vi "UI Style.vi"() -> ()   [LabVIEW 2023, in "VIDoc Parsing.lvlib" / "Structure Reporter.lvlib"]
uses:
  Structure Reporter.lvlib
  <vilib>/platform/TimedLoop/XDataNode/XDataNode.xnode
  <vilib>/Platform/TimedLoop/XDataNode/nitl_modes.ctl
  <vilib>/Platform/TimedLoop/XDataNode/XDNodeRunTimeDep.lvlib
  <vilib>/Platform/TimedLoop/XDataNode/wakeup.ctl
  <vilib>/Platform/TimedLoop/XDataNode/timing_clust.ctl
panel:
  in  "stop":bool
  in  "OK Button":bool
  in  "Boolean":bool
  in  "Numeric":dbl
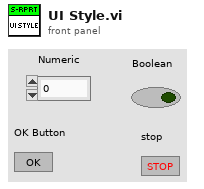
[diagram p1: front panel]
types:
  T1 = typedef "XDNodeRunTimeDep.lvlib/timing_clust.ctl" = cluster{"Expected End [f-1]":u64, "Actual End [f-1]":u64, "Finished Late? [f-1]":bool, "Expected End [i-1]":u64, "Actual End [i-1]":u64, "Finished Late? [i-1]":bool, "Expected Start [i]":u64, "Actual Start [i]":u64, "Expected Start [f]":u64, "Actual Start [f]":u64, "Source Name":string, "Structure Name":string, "Period":i64, "Deadline":i64, "Offset":i64, "Start":i64, "Priority":i32, "Timeout":i32, "Mode":T2, "Wakeup Reason":T3, "Error":errorcluster, "Source Type":string, "Secondary Source Type":string, "Global End Time":u64, "Global Start Time":u64, "Frame Duration":u64, "Iteration Duration":u64, "Assigned CPU":i32, "I/O Scan Engine Mode":u32}
  T2 = typedef "XDNodeRunTimeDep.lvlib/nitl_modes.ctl" = enum32{"No Change", "Process missed periods, maintain original phase", "Discard missed periods, maintain original phase", "Process missed periods, ignore original phase", "Discard missed periods, ignore original phase"}
  T3 = typedef "XDNodeRunTimeDep.lvlib/wakeup.ctl" = enum32{"Normal", "Aborted", "Asynchronous wakeup", "Timing source error", "Timed loop error", "Timeout"}
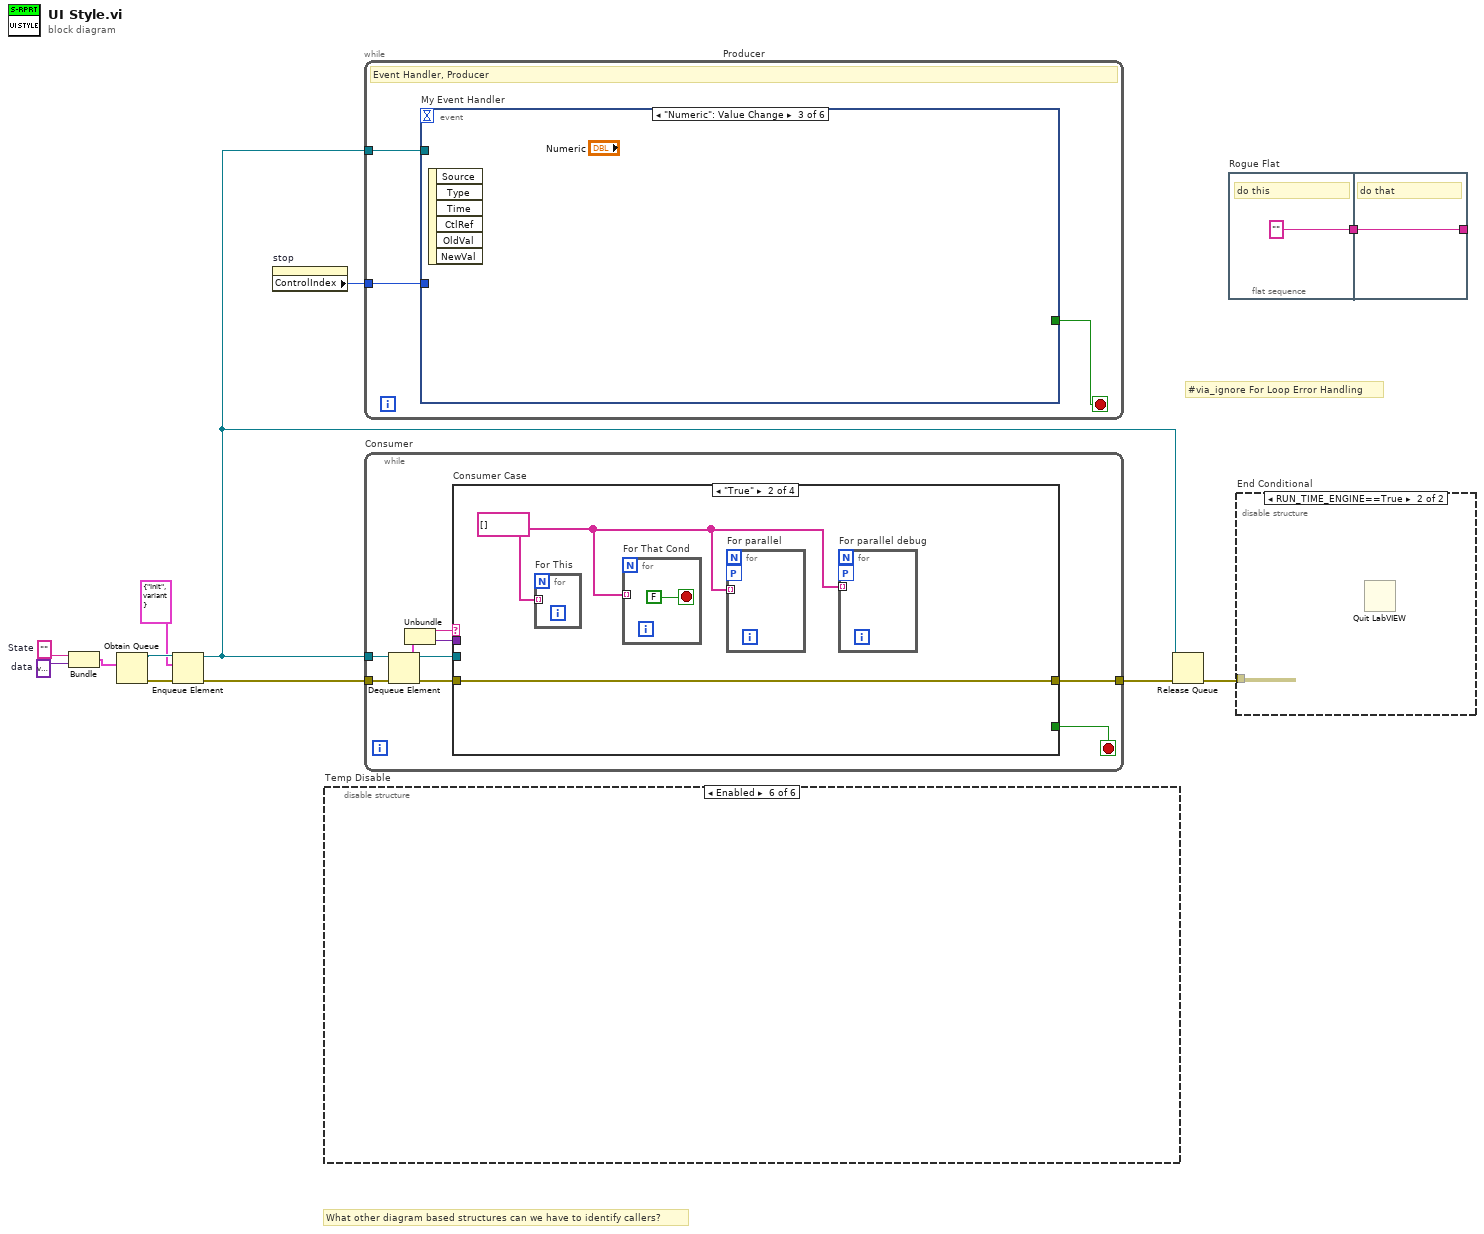
[diagram p0: block diagram]
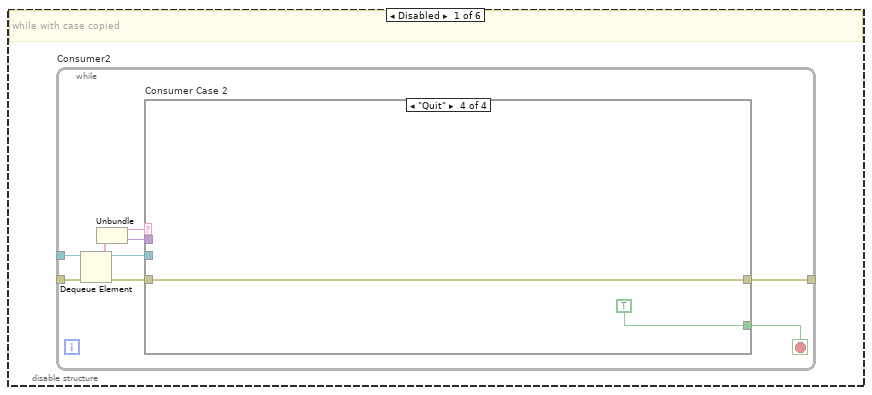
[diagram p3: hidden frame]
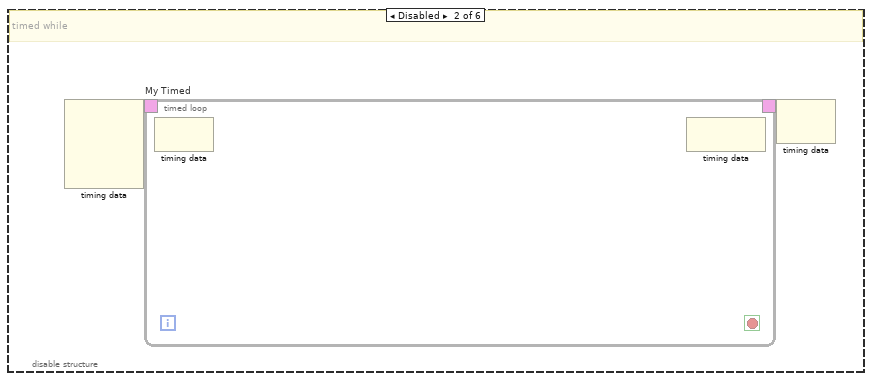
[diagram p7: hidden frame]
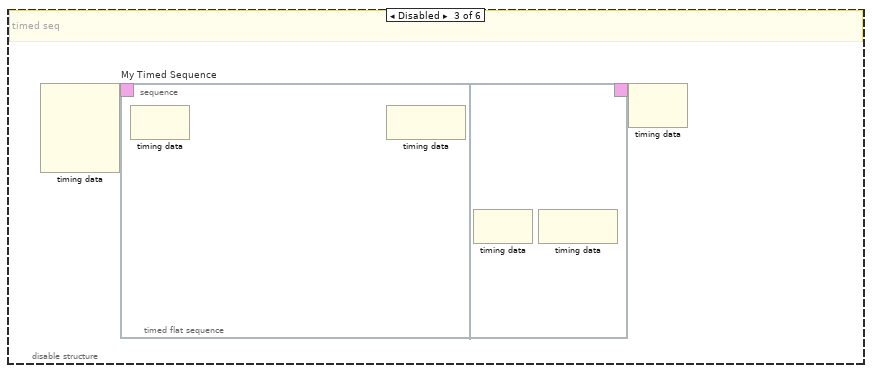
[diagram p8: hidden frame]
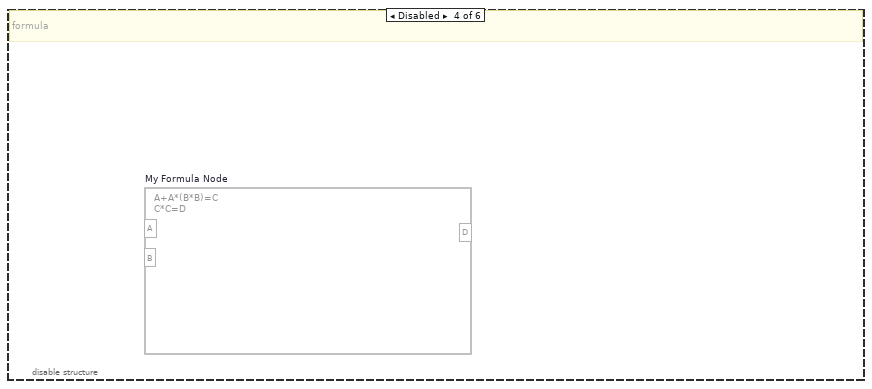
[diagram p9: hidden frame]
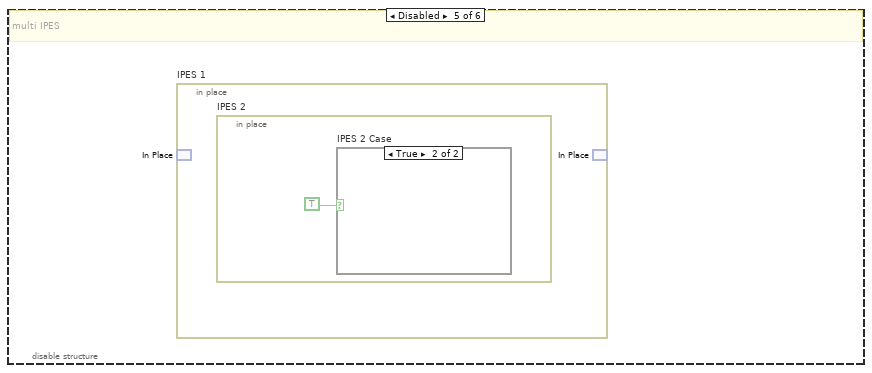
[diagram p10: hidden frame]
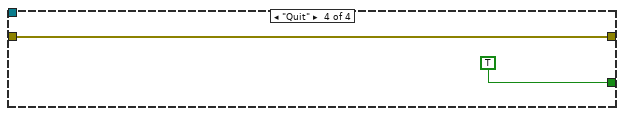
[diagram p14: hidden frame]
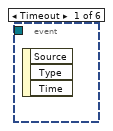
[diagram p15: hidden frame]
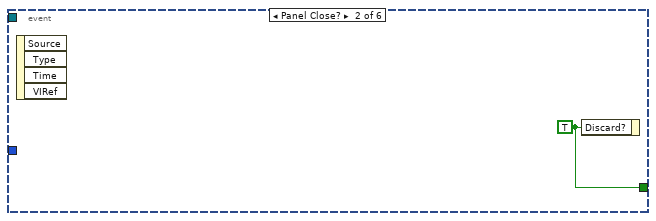
[diagram p16: hidden frame]
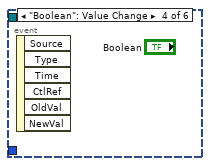
[diagram p17: hidden frame]
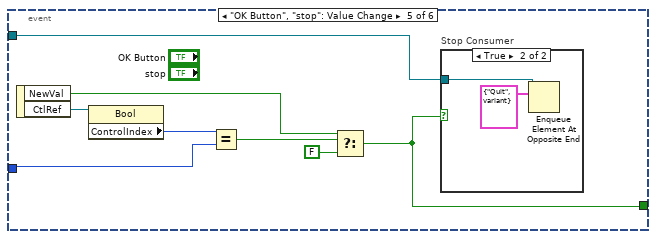
[diagram p18: hidden frame]
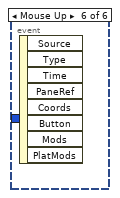
[diagram p20: hidden frame]
diagram:
  w11 = variant  # data
  w12 = ""  # State
  # "#via_ignore For Loop Error Handling"
  # "What other diagram based structures can we have to identify callers?"
  n1 = Bundle("State"=w12, "data"=w11) -> (w10:cluster{"State":string, "data":variant})  [unwired: 1 in]
  n2 = Obtain Queue(element data type=w10) -> (queue out=w9:refnum<queue>, error out=w7:errorcluster)  [unwired: 4 in, 1 out]
  n3 = Enqueue Element(queue=w9, element=cluster{"State":string, "data":variant} {"State"="Init", "data"=variant}, error in (no error)=w7) -> (queue out=w5:refnum<queue>, error out=w8:errorcluster)  [unwired: 1 in, 1 out]
  n4 = property on="stop" class="Bool"() -> ("ControlIndex"=w3:i32)  [unwired: 2 in, 2 out]
  n5 = disable-structure "Temp Disable" shown="Enabled" {
    frame Disabled {
      # "while with case copied"
      n6 = while "Consumer2" {
        tunnel: _ -> [w21]
        tunnel: _ -> [w15]
        tunnel: [w14] -> _
        stop <- w13 stop-if-true
        n7 = Dequeue Element(queue=w21, error in (no error)=w15) -> (queue out=w17:refnum<queue>, element=w20:cluster{"State":string, "data":variant}, error out=w16:errorcluster)  [unwired: 1 in, 1 out]
        n8 = Unbundle(w20) -> ("State"=w19:string, "data"=w18:variant)
        n9 = case "Consumer Case 2" shown="\"Quit\"" w19 {
          tunnel: w18 -> [_ _ _ _]
          tunnel: w17 -> [_ _ _ _]
          tunnel: w16 -> [w22 w23 w24 w29]
          tunnel: [w22 w23 w26 w29] -> w14
          tunnel: [_ _ _ TRUE] -> w13
          frame "False", Default {
          }
          frame "True" {
          }
          frame "Init" {
            n10 = flat-sequence "Init Flat 2" {
              tunnel: [w27] -> w25
              tunnel: w24 -> [w27]
              tunnel: [w28] -> w26
              tunnel: w25 -> [w28]
              frame #0 {
                # "do this"
              }
              frame #1 {
                # "do that"
              }
            }
          }
          frame "Quit" {
          }
        }
      }
    }
    frame Disabled {
      # "timed while"
      n11 = node-c288() -> (w32:T1)  [unwired: 4 in]
      n12 = timed-loop "My Timed" {
        timing: w32 -> [_]
        timing-out: [_] -> w31
        stop <- _ stop-if-true
        n13 = node-c288() -> ()  [unwired: 1 in, 1 out]
        n14 = node-c288() -> ()  [unwired: 1 in, 1 out]
      }
      n15 = node-c288(w31) -> ()  [unwired: 1 out]
    }
    frame Disabled {
      # "timed seq"
      n16 = node-c288() -> (w38:T1)  [unwired: 4 in]
      n17 = timed-sequence "My Timed Sequence" {
        timing: w38 -> [_]
        timing-out: [_] -> w37
        n18 = timed-flat-sequence {
          frame #0 {
            n19 = node-c288() -> ()  [unwired: 1 in, 1 out]
            n20 = node-c288() -> ()  [unwired: 1 in, 1 out]
          }
          frame #1 {
            n21 = node-c288() -> ()  [unwired: 1 in, 1 out]
            n22 = node-c288() -> ()  [unwired: 1 in, 1 out]
          }
        }
      }
      n23 = node-c288(w37) -> ()  [unwired: 1 out]
    }
    frame Disabled {
      # "formula"
      n24 = formula code="A+A*(B*B)=C\nC*C=D" "My Formula Node"() -> ()  [unwired: 2 in, 1 out]
    }
    frame Disabled {
      # "multi IPES"
      n25 = in-place "IPES 1" {
        n26 = in-place-match #1() -> ()  [unwired: 1 in, 1 out]
        n27 = in-place "IPES 2" {
          n28 = case "IPES 2 Case" shown="True" TRUE {
            frame False {
            }
            frame True {
            }
          }
        }
        n29 = in-place-match #1() -> ()  [unwired: 1 in, 1 out]
      }
    }
    frame Enabled {
    }
  }
  n30 = while "Producer" {
    tunnel: w5 -> [w47]
    tunnel: w3 -> [w46]
    stop <- w48 stop-if-true
    # "Event Handler, Producer"
    n31 = event "My Event Handler" shown="[2] \"Numeric\": Value Change" {
      selector: _ -> [_ _ _ _ _ _]
      dyn-events: _ -> [_ _ _ _ _ _]
      timeout: _ -> [_ _ _ _ _ _]
      tunnel: [_ w49 _ _ w51 _] -> w48
      tunnel: w47 -> [_ _ _ _ w50 _]
      tunnel: w46 -> [_ _ _ _ w55 _]
      event Timeout {
        n32 = event-data() -> ()  [unwired: 1 in, 3 out]
      }
      event Panel Close? {
        w49 = TRUE ("Discard?")
        n33 = event-data() -> ()  [unwired: 1 in, 4 out]
        n34 = event-data("Discard?"=w49) -> ()  [unwired: 1 in, 1 out]
      }
      event "Numeric": Value Change {
        n35 = event-data() -> ()  [unwired: 1 in, 6 out]
      }
      event "Boolean": Value Change {
        n36 = event-data() -> ()  [unwired: 1 in, 6 out]
      }
      event "OK Button", "stop": Value Change {
        n37 = event-data() -> ("NewVal"=w53:bool, "CtlRef"=w57:refnum<vi>)  [unwired: 1 in]
        n38 = property class="Bool"(reference=w57) -> ("ControlIndex"=w56:i32)  [unwired: 1 in, 2 out]
        n39 = Equal?(x=w56, y=w55) -> (x = y?=w54:bool)
        n40 = Select(t=w53, s=w54, f=FALSE) -> (s? t:f=w51:bool)
        n41 = case "Stop Consumer" shown="True" w51 {
          tunnel: w50 -> [_ w59]
          frame False {
          }
          frame True {
            n42 = Enqueue Element At Opposite End(queue=w59, element=cluster{"State":string, "data":variant} {"State"="Quit", "data"=variant}) -> ()  [unwired: 2 in, 3 out]
          }
        }
      }
      event Mouse Up {
        n43 = event-data() -> ()  [unwired: 1 in, 8 out]
      }
    }
  }
  n44 = while "Consumer" {
    tunnel: w5 -> [w68]
    tunnel: w8 -> [w62]
    tunnel: [w61] -> w6
    stop <- w60 stop-if-true
    n45 = Dequeue Element(queue=w68, error in (no error)=w62) -> (queue out=w64:refnum<queue>, element=w67:cluster{"State":string, "data":variant}, error out=w63:errorcluster)  [unwired: 1 in, 1 out]
    n46 = Unbundle(w67) -> ("State"=w66:string, "data"=w65:variant)
    n47 = case "Consumer Case" shown="\"True\"" w66 {
      tunnel: w65 -> [_ _ _ _]
      tunnel: w64 -> [_ _ _ _]
      tunnel: w63 -> [w69 w71 w73 w78]
      tunnel: [w69 w71 w75 w78] -> w61
      tunnel: [_ _ _ TRUE] -> w60
      frame "False", Default {
      }
      frame "True" {
        w70 = string[] []
        n48 = for "For This" {
          tunnel: w70 -> [_] mode=indexing
        }
        n49 = for "For That Cond" {
          tunnel: w70 -> [_] mode=indexing
          stop <- FALSE stop-if-true
        }
        n50 = for "For parallel" {
          workers-P: _ -> [_]
          tunnel: w70 -> [_] mode=indexing
        }
        n51 = for "For parallel debug" {
          workers-P: _ -> [_]
          tunnel: w70 -> [_] mode=indexing
        }
      }
      frame "Init" {
        n52 = flat-sequence "Init in order" {
          tunnel: [w76] -> w74
          tunnel: w73 -> [w76]
          tunnel: [w77] -> w75
          tunnel: w74 -> [w77]
          frame #0 {
            # "do this"
          }
          frame #1 {
            # "do that"
          }
        }
      }
      frame "Quit" {
      }
    }
  }
  n53 = Release Queue(queue=w5, error in (no error)=w6) -> (error out=w4:errorcluster)  [unwired: 1 in, 2 out]
  n54 = flat-sequence "Rogue Flat" {
    tunnel: [""] -> w1
    tunnel: w1 -> [w81]
    tunnel: [w81] -> _
    frame #0 {
      # "do this"
    }
    frame #1 {
      # "do that"
    }
  }
  n55 = disable-structure "End Conditional" shown="RUN_TIME_ENGINE==True" {
    disable-tunnel: w4 -> [_ _]
    frame condition #0 (active) {
    }
    frame condition #1 {
      n56 = Quit LabVIEW() -> ()  [unwired: 1 in]
    }
  }
